vi "level2.vi"(7 "reset(F)":bool, 8 "Debounce Period(5000 ms)":u32=5000, 9 "period(0.1s)":dbl=0.1 format="%#_13g", 11 "#Left In Q":dbl) -> (0 "s? t:f":u32, 2 "LogInQ changing Speed(#/s)":dbl, 3 "Enum":T1)   [LabVIEW 2017]
uses:
  user.lib/_NEVSTOP/Communicable State Machine(CSM)/Utility/_support/Periodic String Filter Level.ctl
  user.lib/_NEVSTOP/Communicable State Machine(CSM)/Communicable State Machine.lvlib
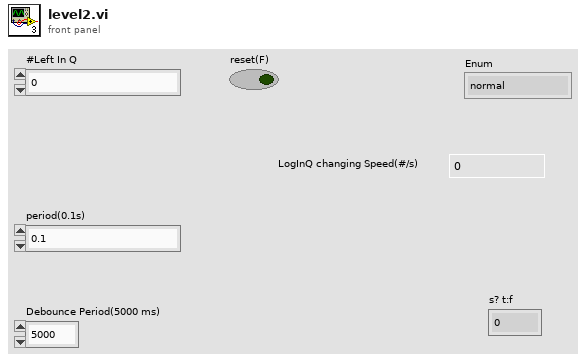
[diagram p1: front panel]
types:
  T1 = typedef "Communicable State Machine.lvlib/Periodic String Filter Level.ctl" = enum16{"normal", "L1", "L2", "L3", "L4"}
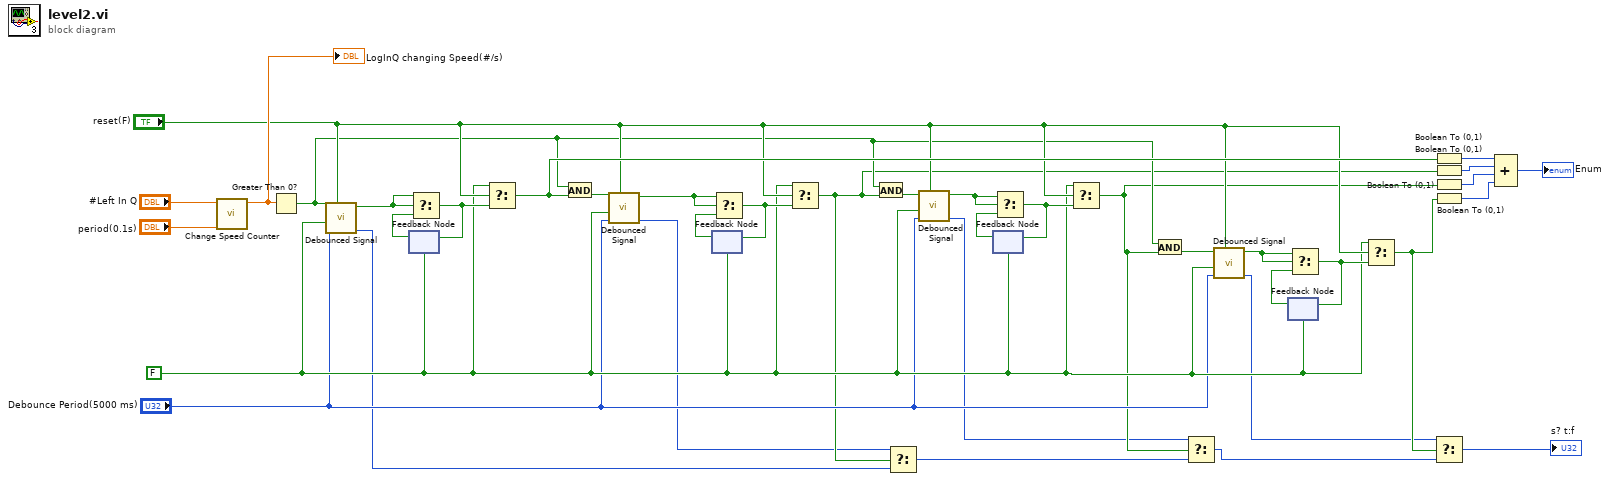
[diagram p0: block diagram]
diagram:
  w17 = FALSE ("reset value")
  n1 = call "Change Speed Counter.vi"("period(0.1s)"="period(0.1s)", "Numeric"="#Left In Q") -> ("Speed(#/s)"=w36:dbl)  [unwired: 7 in, 2 out]
  "LogInQ changing Speed(#/s)" <- w36
  n2 = Greater Than 0?(x=w36) -> (x > 0?=w12:bool)
  n3 = call "Debounced Signal.vi"("reset(F)"="reset(F)", "Debounce Period(ms)"="Debounce Period(5000 ms)", "reset value"=w17, "Signal"=w12) -> ("Since Last Change(ms)"=w8:u32, "signal(safe)"=w37:bool)  [unwired: 6 in]
  n4 = feedback #1(w17) -> (w38:bool)
  n5 = Select(t=w37, s=w37, f=w38) -> (s? t:f=w33:bool)
  n6 = feedback-in #1(w33) -> ()
  n7 = Select(t=w17, s="reset(F)", f=w33) -> (s? t:f=w26:bool)
  n8 = And(x=w12, y=w26) -> (x .and. y?=w15:bool)
  n9 = call "Debounced Signal.vi"("reset(F)"="reset(F)", "Debounce Period(ms)"="Debounce Period(5000 ms)", "reset value"=w17, "Signal"=w15) -> ("Since Last Change(ms)"=w9:u32, "signal(safe)"=w30:bool)  [unwired: 6 in]
  n10 = feedback #2(w17) -> (w31:bool)
  n11 = Select(t=w30, s=w30, f=w31) -> (s? t:f=w32:bool)
  n12 = feedback-in #2(w32) -> ()
  n13 = Select(t=w17, s="reset(F)", f=w32) -> (s? t:f=w10:bool)
  n14 = And(x=w12, y=w10) -> (x .and. y?=w14:bool)
  n15 = Select(t=w9, s=w10, f=w8) -> (s? t:f=w5:u32)
  n16 = call "Debounced Signal.vi"("reset(F)"="reset(F)", "Debounce Period(ms)"="Debounce Period(5000 ms)", "reset value"=w17, "Signal"=w14) -> ("Since Last Change(ms)"=w6:u32, "signal(safe)"=w27:bool)  [unwired: 6 in]
  n17 = feedback #3(w17) -> (w29:bool)
  n18 = Select(t=w27, s=w27, f=w29) -> (s? t:f=w28:bool)
  n19 = feedback-in #3(w28) -> ()
  n20 = Select(t=w17, s="reset(F)", f=w28) -> (s? t:f=w7:bool)
  n21 = And(x=w12, y=w7) -> (x .and. y?=w13:bool)
  n22 = Select(t=w6, s=w7, f=w5) -> (s? t:f=w2:u32)
  n23 = call "Debounced Signal.vi"("reset(F)"="reset(F)", "Debounce Period(ms)"="Debounce Period(5000 ms)", "reset value"=w17, "Signal"=w13) -> ("Since Last Change(ms)"=w3:u32, "signal(safe)"=w21:bool)  [unwired: 6 in]
  n24 = feedback #4(w17) -> (w19:bool)
  n25 = Select(t=w21, s=w21, f=w19) -> (s? t:f=w20:bool)
  n26 = feedback-in #4(w20) -> ()
  n27 = Select(t=w17, s="reset(F)", f=w20) -> (s? t:f=w4:bool)
  n28 = Boolean To (0,1)(Boolean=w26) -> (0, 1=w25:i16)
  n29 = Boolean To (0,1)(Boolean=w10) -> (0, 1=w24:i16)
  n30 = Boolean To (0,1)(Boolean=w7) -> (0, 1=w23:i16)
  n31 = Boolean To (0,1)(Boolean=w4) -> (0, 1=w16:i16)
  n32 = Select(t=w3, s=w4, f=w2) -> (s? t:f=→"s? t:f":u32)
  n33 = Compound Arithmetic op=ADD(w25, w24, w23, w16) -> (→"Enum":i16)
